vi "Unit Test Allow Parent Level Removed False.vi"() -> ()   [LabVIEW 2019, in "Sports Unit Tests.lvclass"]
uses:
  Sports Unit Tests.lvclass
  Classes/Kareem Abdul-Jabbar/Kareem Abdul-Jabbar.lvclass
  <userlib>/Blue Origin/BlueSerialization/BlueSerializer/DeserializeOptions.ctl
  <userlib>/Blue Origin/BlueSerialization/BlueSerializer/DeserializeSlicingOptions.ctl
  <userlib>/Blue Origin/BlueSerialization/BlueSerializer/DeserializeMutationOptions.ctl
  <userlib>/Blue Origin/BlueSerialization/BlueSerializer/DeserializePreservationOptions.ctl
  <userlib>/Blue Origin/BlueSerialization/BlueSerializer/PreserveNonWiredDataOption.ctl
  <vilib>/Utility/error.llb/Clear Errors.vi
  <vilib>/addons/_JKI Toolkits/Caraya/classes/Test/Define Test.vi
  <vilib>/addons/_JKI Toolkits/Caraya/classes/Assert/Assert Equal Value_Variant.vi
  <vilib>/addons/_JKI Toolkits/Caraya/classes/Assert/Assert Error.vi
  <vilib>/addons/_JKI Toolkits/Caraya/classes/Assert/Assert.lvclass
  <userlib>/Blue Origin/BlueSerialization/BlueSerializer/BlueSerializer.lvclass
panel:
  out "Table":string[][](table)=[["{\r  \"Class\":[\"Kareem Abdul-Jabbar.lvclass\",\"Basketball Player.lvclass\",\"Sports Player.lvclass\",\"Human.lvclass\",\"BlueSerialization.lvlib:BlueSerializable.lvclass\"],\r  \"Version\":[\"2.0.0.3\",\"2.0.0.3\",\"2.0.0.3\",\"2.0.0.3\",\"2.0.0.0\"],\r  \"BlueSerialization.lvlib:BlueSerializable.lvclass\":{\"LibVersion\":1},\r  \"Human.lvclass\":{\r    \"alive?\":true,\r    \"Age (years)\":40,\r    \"Name\":\"Shauille O'Neal\",\r    \"Height (ft)\":6\r  },\r  \"Sports Player.lvclass\":{\r    \"Professional?\":true,\r    \"Earnings (dollars)\":1000000,\r    \"Sponsor\":\"Aladin\"\r  },\r  \"Basketball Player.lvclass\":{\r    \"Sports team\":\"Lakers\",\r    \"Free-throw percentage\":99\r  },\r  \"Kareem Abdul-Jabbar.lvclass\":{\"Nickname\":\"Jabberwalkie\"}\r}", "{\r  \"Class\":[\"Kareem Abdul-Jabbar.lvclass\",\"Basketball Player.lvclass\",\"Sports Player.lvclass\",\"Human.lvclass\",\"BlueSerialization.lvlib:BlueSerializable.lvclass\"],\r  \"Version\":[\"2.0.0.3\",\"2.0.0.3\",\"2.0.0.3\",\"2.0.0.3\",\"2.0.0.0\"],\r  \"BlueSerialization.lvlib:BlueSerializable.lvclass\":{\"LibVersion\":1},\r  \"Human.lvclass\":{\r    \"alive?\":true,\r    \"Age (years)\":40,\r    \"Name\":\"Shauille O'Neal\",\r    \"Height (ft)\":6\r  },\r  \"Sports Player.lvclass\":{\r    \"Professional?\":true,\r    \"Earnings (dollars)\":1000000,\r    \"Sponsor\":\"Aladin\"\r  },\r  \"Basketball Player.lvclass\":{\r    \"Sports team\":\"Lakers\",\r    \"Free-throw percentage\":99\r  },\r  \"Kareem Abdul-Jabbar.lvclass\":{\"Nickname\":\"Jabberwalkie\"}\r}", "Status: FALSE\ncode: 0\n", "BlueJSONTextSerializer.lvlib:BlueJSONTextSerializer.lvclass"], ["Class = [\"Kareem Abdul-Jabbar.lvclass\", \"Basketball Player.lvclass\", \"Sports Player.lvclass\", \"Human.lvclass\", \"BlueSerialization.lvlib:BlueSerializable.lvclass\"]\r\nVersion = [\"2.0.0.3\", \"2.0.0.3\", \"2.0.0.3\", \"2.0.0.3\", \"2.0.0.0\"]\r\n\n[\"BlueSerialization.lvlib:BlueSerializable.lvclass\"]\nLibVersion = 1\r\n\n[\"Human.lvclass\"]\n\"alive?\" = true\r\n\"Age (years)\" = 40\r\nName = \"Shauille O'Neal\"\r\n\"Height (ft)\" = 6.0\r\n\n[\"Sports Player.lvclass\"]\n\"Professional?\" = true\r\n\"Earnings (dollars)\" = 1000000.0\r\nSponsor = \"Aladin\"\r\n\n[\"Basketball Player.lvclass\"]\n\"Sports team\" = \"Lakers\"\r\n\"Free-throw percentage\" = 99.0\r\n\n[\"Kareem Abdul-Jabbar.lvclass\"]\nNickname = \"Jabberwalkie\"\r\n", "Class = [\"Kareem Abdul-Jabbar.lvclass\", \"Basketball Player.lvclass\", \"Sports Player.lvclass\", \"Human.lvclass\", \"BlueSerialization.lvlib:BlueSerializable.lvclass\"]\r\nVersion = [\"2.0.0.3\", \"2.0.0.3\", \"2.0.0.3\", \"2.0.0.3\", \"2.0.0.0\"]\r\n\n[\"BlueSerialization.lvlib:BlueSerializable.lvclass\"]\nLibVersion = 1\r\n\n[\"Human.lvclass\"]\n\"alive?\" = true\r\n\"Age (years)\" = 40\r\nName = \"Shauille O'Neal\"\r\n\"Height (ft)\" = 6.0\r\n\n[\"Sports Player.lvclass\"]\n\"Professional?\" = true\r\n\"Earnings (dollars)\" = 1000000.0\r\nSponsor = \"Aladin\"\r\n\n[\"Basketball Player.lvclass\"]\n\"Sports team\" = \"Lakers\"\r\n\"Free-throw percentage\" = 99.0\r\n\n[\"Kareem Abdul-Jabbar.lvclass\"]\nNickname = \"Jabberwalkie\"\r\n", "Status: FALSE\ncode: 0\n", "BlueTOMLSerializer.lvlib:BlueTOMLSerializer.lvclass"]]
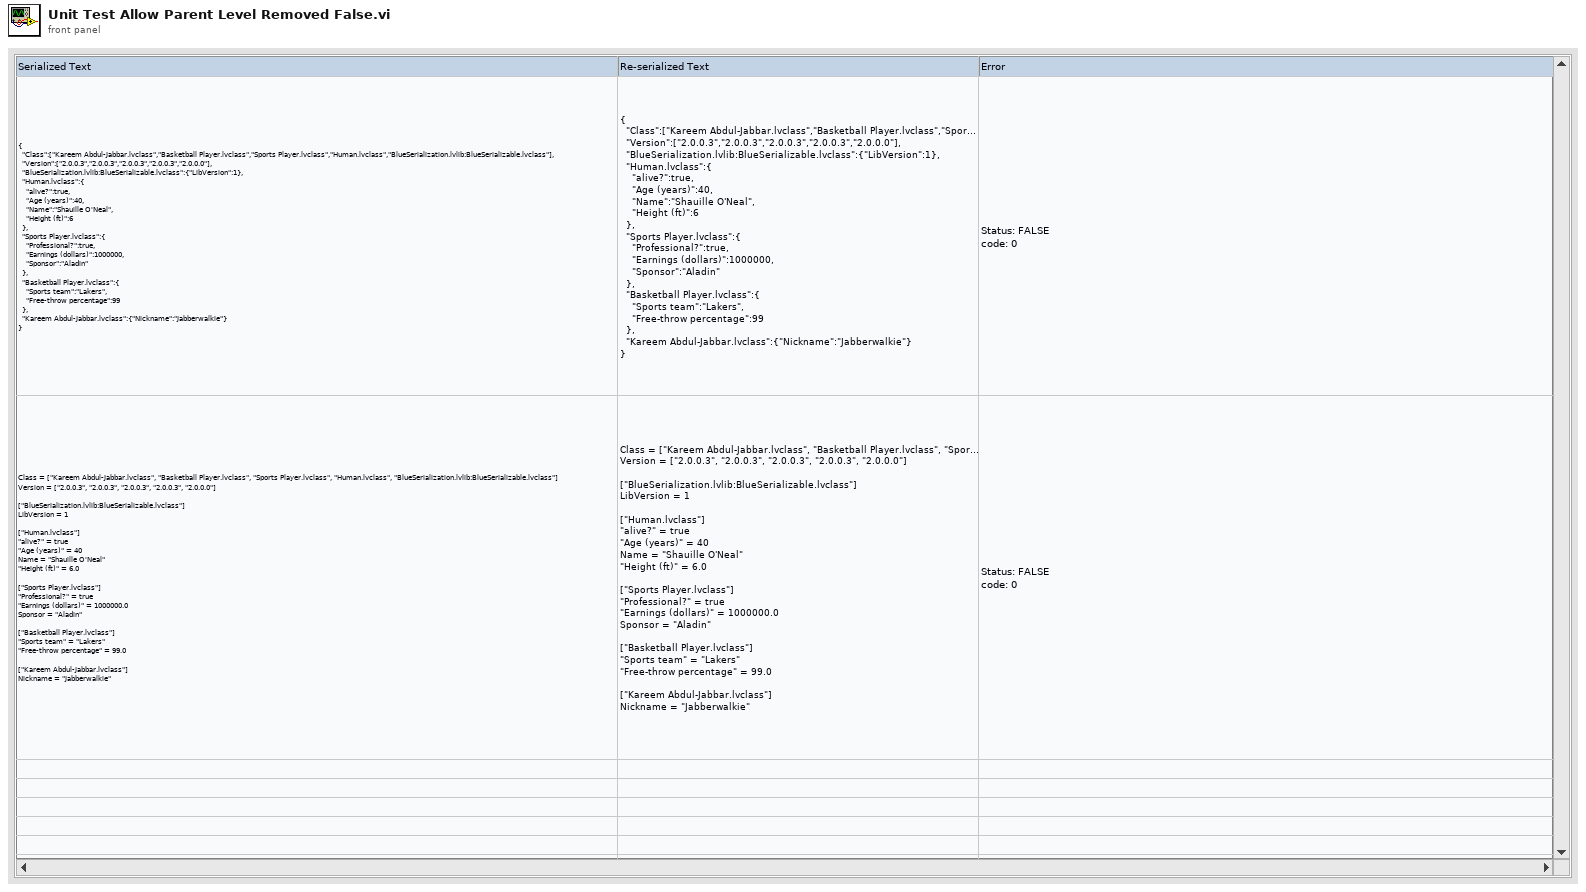
[diagram p1: front panel]
types:
  T1 = typedef "BlueSerialization.lvlib/BlueSerializer.lvclass/DeserializeOptions.ctl" = cluster{"deserialize non-BlueSerializable objects from hex?":bool, "expand objects on type conflict?":bool, "Slicing":T2, "Mutation Options":T3, "Preservation Options":T4}
  T2 = typedef "BlueSerialization.lvlib/BlueSerializer.lvclass/DeserializeSlicingOptions.ctl" = cluster{"slice flattened object data on error?":bool, "sliceable class names":string[]}
  T3 = typedef "BlueSerialization.lvlib/BlueSerializer.lvclass/DeserializeMutationOptions.ctl" = cluster{"error on inserted parent levels?":bool, "\terror on obsolete parent levels?":bool}
  T4 = typedef "BlueSerialization.lvlib/BlueSerializer.lvclass/DeserializePreservationOptions.ctl" = cluster{"Preserve wired serialized data?":bool, "Preserve wired non-serialized data":T5}
  T5 = typedef "BlueSerialization.lvlib/BlueSerializer.lvclass/PreserveNonWiredDataOption.ctl" = enum16{"Don't preserve", "Preserve (error on less-specific wired types)", "Preserve (except on less-specific wired types)"}
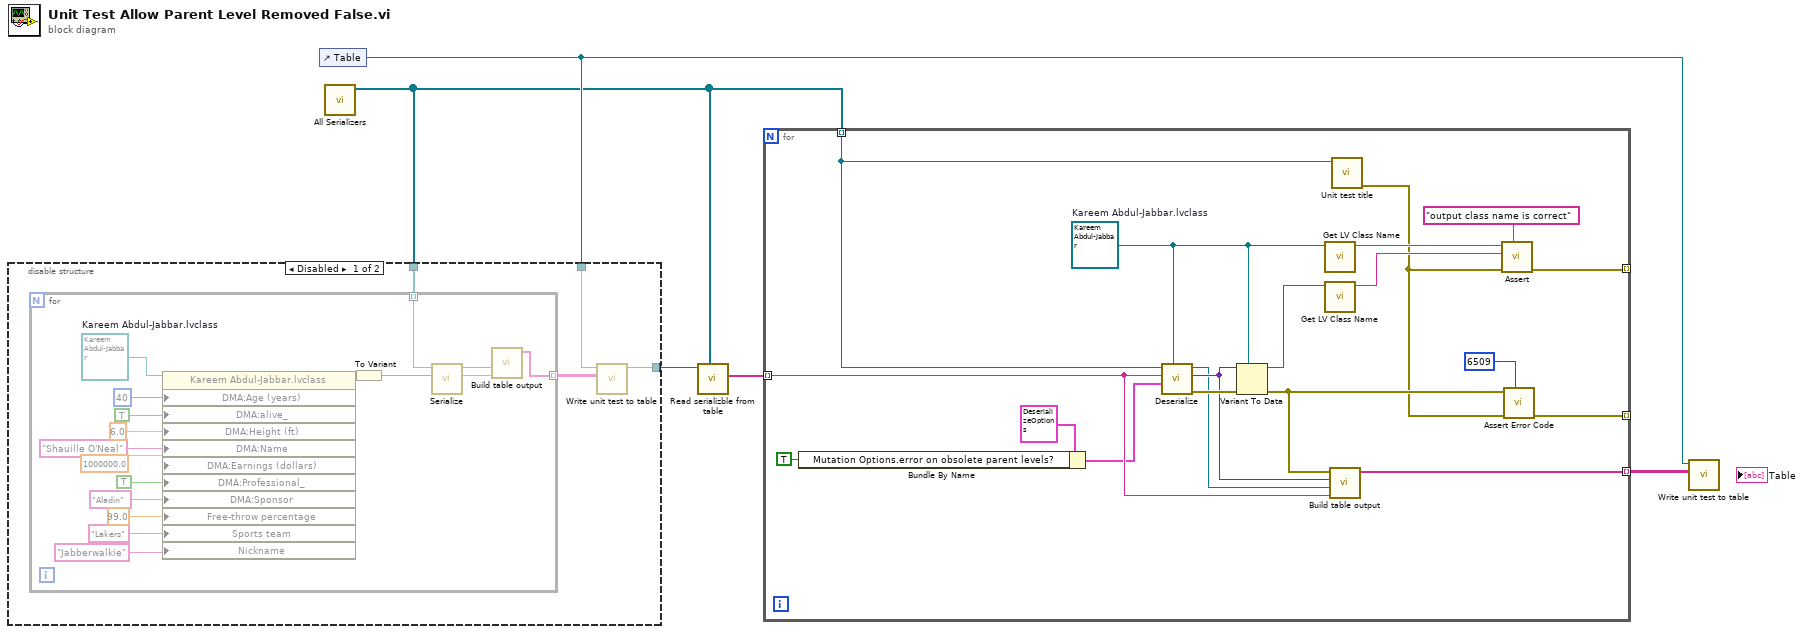
[diagram p0: block diagram]
diagram:
  n1 = control-ref of="Table"() -> (w5:refnum<vi>)
  n2 = call "All Serializers.vi"() -> ("All serializers"=w2:refnum<class "BlueSerializer.lvclass">[])  [unwired: 11 in]
  n3 = disable-structure shown="Disabled" {
    disable-tunnel: w5 -> [w8 w27]
    disable-tunnel: [w7 w27] -> w4
    disable-tunnel: w2 -> [w6 _]
    frame Disabled {
      n4 = for {
        tunnel: w6 -> [w17] mode=indexing
        tunnel: [w14] -> w9 mode=indexing
        w13 = refnum<class "Kareem Abdul-Jabbar.lvclass"> refnum  # Kareem Abdul-Jabbar.lvclass
        n5 = property on="Property Node" class="Kareem Abdul-Jabbar.lvclass"(reference=w13, "DMA:Age (years)"=u16 40 ("Age (years)"), "DMA:alive_"=TRUE ("alive_"), "DMA:Height (ft)"=6.0 ("Height (ft)"), "DMA:Name"="Shauille O'Neal" ("Name"), "DMA:Earnings (dollars)"=1000000.0 ("Earnings (dollars)"), "DMA:Professional_"=TRUE ("Professional_"), "DMA:Sponsor"="Aladin" ("Sponsor"), "Free-throw percentage"=99.0, "Sports team"="Lakers", "Nickname"="Jabberwalkie") -> (reference out=w26:refnum<class "Kareem Abdul-Jabbar.lvclass">)  [unwired: 1 in, 1 out]
        n6 = To Variant(anything=w26) -> (Variant=w18:variant)
        n7 = call <userlib>:"Serialize.vi"("Anything"=w18, "BlueSerializer in"=w17) -> ("Serialized Text"=w16:string, "BlueSerializer out"=w15:refnum<class "BlueSerializer.lvclass">)  [unwired: 7 in, 1 out]
        n8 = call "Build table output.vi"("serialized text"=w16, "BlueSerializer in"=w15) -> ("table output"=w14:string[])  [unwired: 9 in]
      }
      n9 = call "Write unit test to table.vi"("Table"=w9, "Table ref in"=w8) -> ("Table ref out"=w7:refnum<vi>)  [unwired: 9 in]
    }
    frame Enabled {
    }
  }
  n10 = call "Read serializble from table.vi"("serializers"=w2, "Table ref in"=w4) -> ("serializable texts"=w3:string[])  [unwired: 7 in, 2 out]
  n11 = for {
    tunnel: w2 -> [w28] mode=indexing
    tunnel: [w33] -> _ mode=indexing
    tunnel: [w41] -> _ mode=indexing
    tunnel: w3 -> [w38] mode=indexing
    tunnel: [w37] -> w1 mode=indexing
    w36 = refnum<class "Kareem Abdul-Jabbar.lvclass"> refnum  # Kareem Abdul-Jabbar.lvclass
    n12 = Bundle By Name(cluster=T1 {"deserialize non-BlueSerializable objects from hex?"=FALSE, "expand objects on type conflict?"=FALSE, "Slicing"={"slice flattened object data on error?"=FALSE, "sliceable class names"=[]}, "Mutation Options"={"error on inserted parent levels?"=FALSE, "\terror on obsolete parent levels?"=FALSE}, "Preservation Options"={"Preserve wired serialized data?"=FALSE, "Preserve wired non-serialized data"=enum."Don't preserve"}} ("Deserialize Options"), "Mutation Options.error on obsolete parent levels?"=TRUE ("Allow class expansion?")) -> (w29:T1)
    n13 = call <userlib>:"Deserialize.vi"("Anything"=w36, "Deserialize Options"=w29, "Serialized Text"=w38, "BlueSerializer in"=w28) -> ("error out"=w46:errorcluster, "Variant"=w40:variant, "BlueSerializer out"=w39:refnum<class "BlueSerializer.lvclass">)  [unwired: 5 in]
    n14 = Variant To Data(error in=w46, type=w36, Variant=w40) -> (data=w45:refnum<class "Kareem Abdul-Jabbar.lvclass">, error out=w35:errorcluster)
    n15 = call <vilib>:"Get LV Class Name.vi"("object"=w36) -> ("class name"=w44:string)  [unwired: 9 in, 1 out]
    n16 = call <vilib>:"Get LV Class Name.vi"("object"=w45) -> ("class name"=w43:string)  [unwired: 9 in, 1 out]
    n17 = call "Build table output.vi"("serialized text"=w38, "BlueSerializer in"=w39, "deserialized variant"=w40, "variant to data error"=w35) -> ("table output"=w37:string[])  [unwired: 7 in]
    n18 = call "Unit test title.vi"("serializer"=w28) -> ("error out"=w34:errorcluster)  [unwired: 9 in, 1 out]
    n19 = call-poly <vilib>:"Assert.vi"("Label"="output class name is correct", "error in (no error)"=w34, "Y"=w43, "X"=w44) -> ("error out"=w41:errorcluster)  [unwired: 7 in]
    n20 = call "Assert Error Code.vi"("Assert specific error code"=6509, "error in (no error)"=w34, "Error?"=w35) -> ("error out"=w33:errorcluster)  [unwired: 8 in]
  }
  n21 = call "Write unit test to table.vi"("Table"=w1, "Table ref in"=w5) -> ()  [unwired: 9 in, 1 out]
